vi "Get Compiled Inline Async Settings.vi"(8 "error in":errorcluster, 11 "Variant":variant) -> (0 "error out":errorcluster, 3 "Compiled Inline Async Settings":T1 {"Read"."Refs"."Data Reference" format="%.0x"; "Write"."Refs"."Data Reference" format="%.0x"; "ReadWrite"."Refs" format="%.0x"})   [LabVIEW 2026, in "Template Debug Tools.lvlib"]
uses:
  Template Debug Tools.lvlib
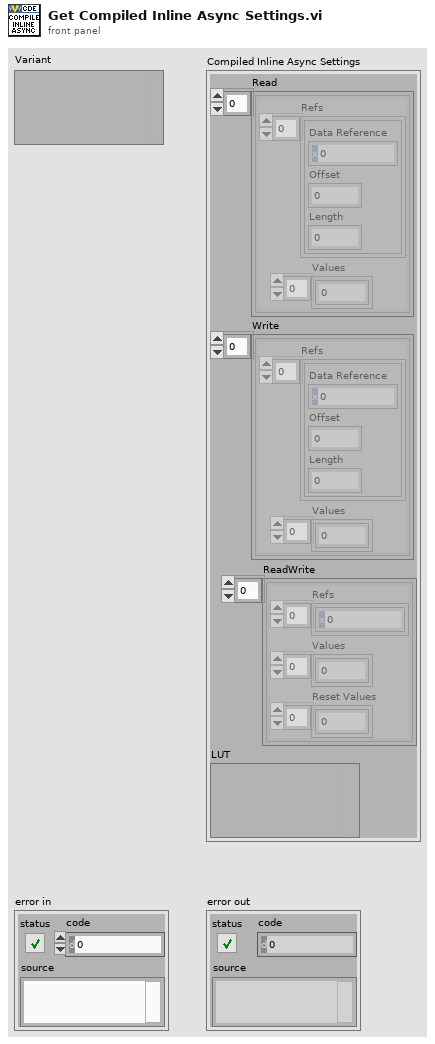
[diagram p1: front panel]
types:
  T1 = cluster{"Read":cluster{"Refs":cluster{"Data Reference":i32, "Offset":u64, "Length":u64}[], "Values":dbl[]}[], "Write":cluster{"Refs":cluster{"Data Reference":i32, "Offset":u64, "Length":u64}[], "Values":dbl[]}[], "ReadWrite":cluster{"Refs":i32[], "Values":dbl[], "Reset Values":dbl[]}[], "LUT":variant}
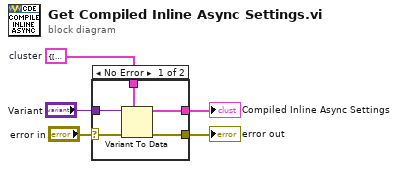
[diagram p0: block diagram]
diagram:
  w4 = T1 {"Read"=[], "Write"=[], "ReadWrite"=[], "LUT"=variant}  # cluster
  n1 = case shown="No Error" "error in" {
    selector: "error in" -> [w6 w12]
    tunnel: "Variant" -> [w10 _]
    tunnel: w4 -> [w9 w11]
    tunnel: [w8 w11] -> w3
    tunnel: [w7 w12] -> w2
    frame No Error {
      n2 = Variant To Data(error in=w6, type=w9, Variant=w10) -> (data=w8:T1, error out=w7:errorcluster)
    }
    frame Error {
    }
  }
  "Compiled Inline Async Settings" <- w3
  "error out" <- w2
